vi "Refresh.vi"(8 "error in (no error)":errorcluster, 11 "Pane Relief Main UI in":refnum<class "Pane Relief Main UI.lvclass">) -> (0 "error out":errorcluster, 3 "Pane Relief Main UI out":refnum<class "Pane Relief Main UI.lvclass">)   [LabVIEW 2015, in "Pane Relief Main UI.lvlib" / "Pane Relief Main UI.lvclass"]
uses:
  Pane Relief Main UI.lvclass
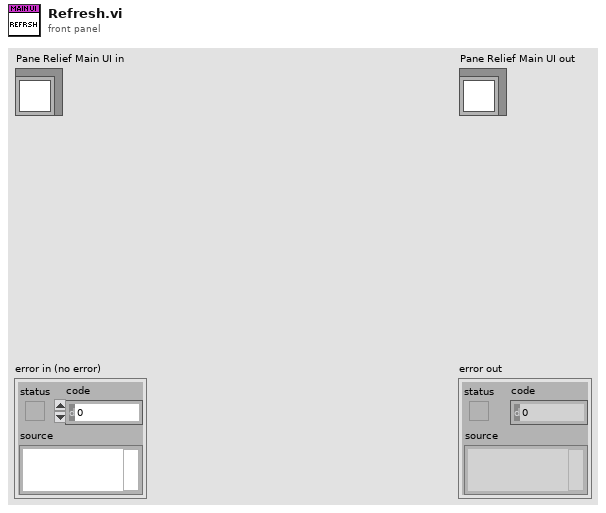
[diagram p1: front panel]
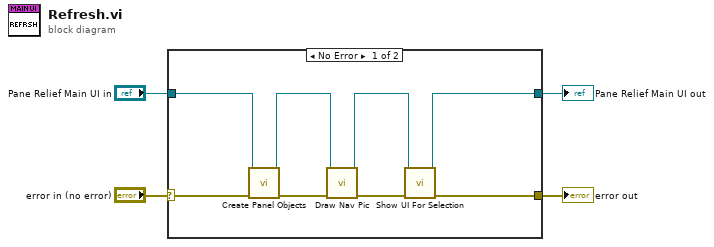
[diagram p0: block diagram]
diagram:
  n1 = case shown="No Error" "error in (no error)" {
    selector: "error in (no error)" -> [w8 w14]
    tunnel: [w7 w14] -> w3
    tunnel: [w5 w13] -> w1
    tunnel: "Pane Relief Main UI in" -> [w6 w13]
    frame No Error {
      n2 = call-dynamic "Create Panel Objects.vi"("Error In"=w8, "Pane Relief Main UI in"=w6) -> ("Error Out"=w11:errorcluster, "Pane Relief Main UI out"=w12:refnum<class "Pane Relief Main UI.lvclass">)  [unwired: 8 in]
      n3 = call-dynamic "Draw Nav Pic.vi"("Error In"=w11, "Pane Relief Main UI in"=w12) -> ("Error Out"=w9:errorcluster, "Pane Relief Main UI out"=w10:refnum<class "Pane Relief Main UI.lvclass">)  [unwired: 8 in]
      n4 = call-dynamic "Show UI For Selection.vi"("Error In"=w9, "Pane Relief Main UI in"=w10) -> ("Error Out"=w7:errorcluster, "Pane Relief Main UI out"=w5:refnum<class "Pane Relief Main UI.lvclass">)  [unwired: 8 in]
    }
    frame Error {
    }
  }
  "error out" <- w3
  "Pane Relief Main UI out" <- w1
